vi "PCI1220U退出.vi"(10 "DeviceHandle IN":u32, 11 "AxisHandle IN":u32) -> ()   [LabVIEW 2011]
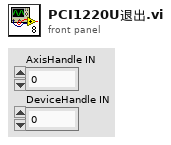
[diagram p1: front panel]
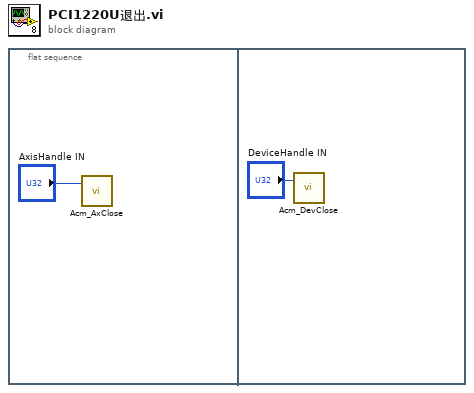
[diagram p0: block diagram]
diagram:
  n1 = flat-sequence {
    frame #0 {
      n2 = call <userlib>:"Acm_AxClose.vi"("AxisHandle"="AxisHandle IN") -> ()  [unwired: 1 in, 2 out]
    }
    frame #1 {
      n3 = call <userlib>:"Acm_DevClose.vi"("DeviceHandle"="DeviceHandle IN") -> ()  [unwired: 1 in, 2 out]
    }
  }
